vi "matlabtest.vi"() -> ()   [LabVIEW 2015]
uses:
  <vilib>/imath/engines/lvmath2/RunTimeEngine/Managers/WorkSpace/UID Generator.vi
  \\hs1.lboro.ac.uk\eljsl/LabVIEW Data/MathScriptVIs/MCStatic_35235434032_815edb1f09f148c670391748a9bc2594.vi
  <instcachedir>/0/MCStatic_35235434032_815edb1f09f148c670391748a9bc2594_4564CBA6A3C349568B155A0F362F05A2.lvgen/MCStatic_35235434032_815edb1f09f148c670391748a9bc2594_4564CBA6A3C349568B155A0F362F05A2_000.vi
  <vilib>/imath/engines/lvmath2/RunTimeEngine/RunTimeType/NIMS_RunTimeType_From StrictType (excl LVString).vi
  <instcachedir>/0/NIMS_RunTimeType_From StrictType (excl LVString)_EB1C38A9BC5048DA9ABDA8F781E54D21.lvgen/NIMS_RunTimeType_From StrictType (excl LVString)_EB1C38A9BC5048DA9ABDA8F781E54D21_000.vi
  <vilib>/imath/engines/lvmath2/RunTimeEngine/LocalVariableDefStatement/MC_LocalVariableDefStatement_Display.vi
  <vilib>/imath/engines/lvmath2/RunTimeEngine/Managers/SymbolTable/Clear UID.vi
  <vilib>/imath/engines/lvmath2/RunTimeEngine/NodeEndStatement/NIMS_NodeEndStatement_Output.vi
  <instcachedir>/0/NIMS_NodeEndStatement_Output_53EC0D466D134D7ABD903AC30B43404B.lvgen/NIMS_NodeEndStatement_Output_53EC0D466D134D7ABD903AC30B43404B_010.vi
  <vilib>/imath/engines/lvmath2/RunTimeEngine/ErrorHandling/NIMS_Finalize Error.vi
  f_1.m
  <vilib>/imath/engines/lvmath2/RunTimeEngine/Managers/SymbolTable/NIMS_WorkSpace.lvlib
panel:
  out "x":i32
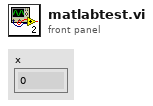
[diagram p1: front panel]
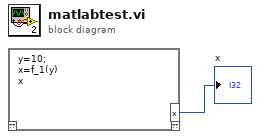
[diagram p0: block diagram]
diagram:
  n1 = mathscript code="y=10;\nx=f_1(y)\nx"() -> ("x"=→"x":i32)  [unwired: 1 in, 1 out]
